vi "autofocus-view-calibration.vi"() -> ()   [LabVIEW 2014]
uses:
  autofocus-globals.vi
  TIRF/tirf-lock-globals.vi
panel:
  out "XY Graph":cluster{"Y":dbl[], "Y":dbl[]}[](graph)
  in  "Display":bool=TRUE
  out "Calibration curve":cluster{ext[], dbl[]}(graph)
  in  "?":bool
  in  "stop":bool
  out "Intensity 2":cluster{"X position":dbl, "Y position":dbl}(graph)
  out "Power Intensity":dbl(graph)
  # "Divide \nBy Sum"
  # "Raw"
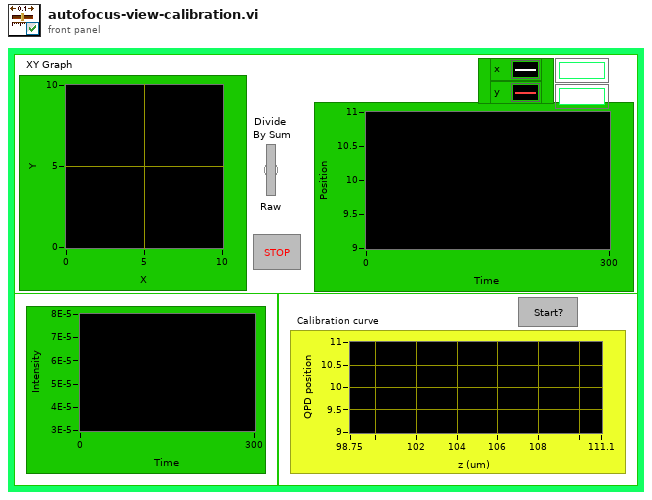
[diagram p1: front panel]
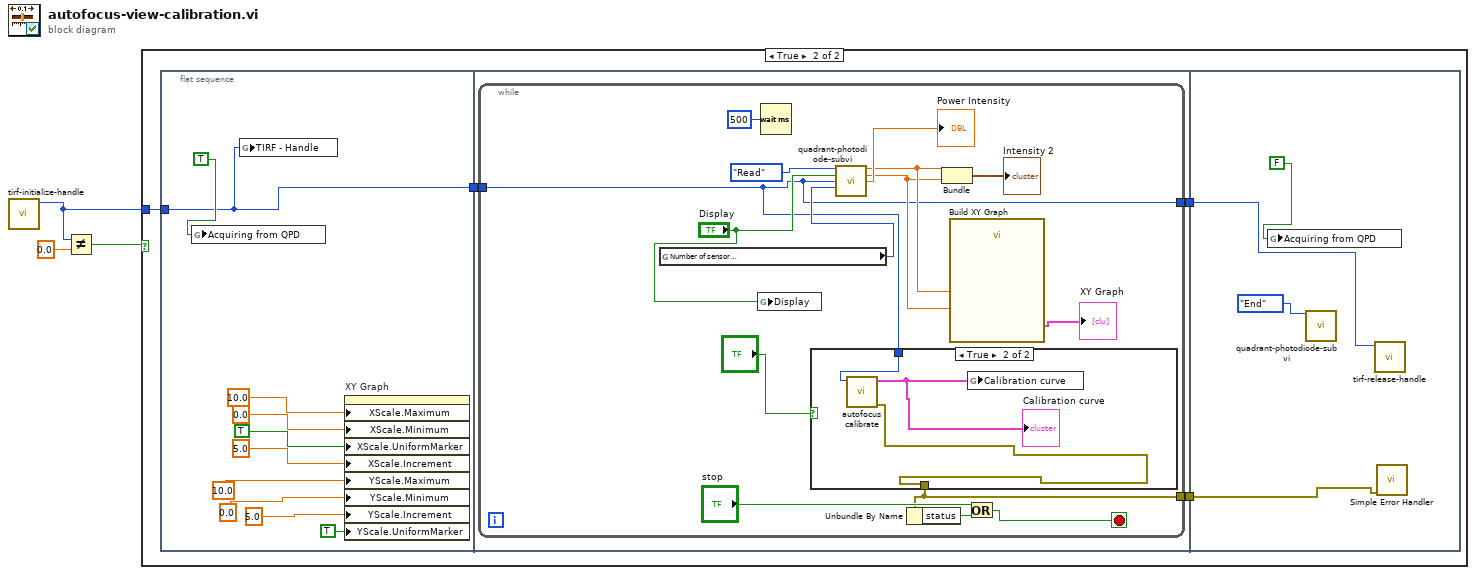
[diagram p0: block diagram]
diagram:
  n1 = call "tirf-initialize-handle.vi"() -> ("handle"=w1:i32)  [unwired: 11 in]
  n2 = Not Equal?(x=w1, y=0.0) -> (x != y?=w2:bool)
  n3 = case shown="True" w2 {
    tunnel: w1 -> [_ w5]
    frame False {
    }
    frame True {
      n4 = flat-sequence {
        tunnel: [w16] -> w6
        tunnel: w5 -> [w16]
        tunnel: [w20] -> w7
        tunnel: w6 -> [w19]
        tunnel: [w18] -> w4
        tunnel: w7 -> [w39]
        tunnel: w4 -> [w40]
        frame #0 {
          n5 = global write "autofocus-globals.vi" "Acquiring from QPD"(TRUE) -> ()
          n6 = global write "autofocus-globals.vi" "TIRF - Handle"(w16) -> ()
          n7 = property on="XY Graph" class="XYGraph (strict)"("XScale.Maximum"=10.0 ("X Scale.Range:Maximum"), "XScale.Minimum"=0.0 ("X Scale.Range:Minimum"), "XScale.UniformMarker"=TRUE ("X Scale.Uniform Marker Spacing?"), "XScale.Increment"=5.0 ("X Scale.Range:Increment"), "YScale.Maximum"=10.0 ("Y Scale.Range:Maximum"), "YScale.Minimum"=0.0 ("Y Scale.Range:Minimum"), "YScale.Increment"=5.0 ("Y Scale.Range:Increment"), "YScale.UniformMarker"=TRUE ("Y Scale.Uniform Marker Spacing?")) -> ()  [unwired: 2 in, 2 out]
        }
        frame #1 {
          n8 = while {
            tunnel: [w25] -> w20
            tunnel: w19 -> [w22]
            tunnel: [w22] -> w18
            stop <- w26 stop-if-true
            n9 = global read "autofocus-globals.vi" "Number of sensor\nreadings to average"() -> (w24:i32)
            n10 = global write "tirf-lock-globals.vi" "Display"("Display") -> ()
            n11 = Wait (ms)(milliseconds to wait=u32 500) -> ()  [unwired: 1 out]
            n12 = case shown="True" "?" {
              tunnel: [_ w37] -> w25
              tunnel: w22 -> [_ w38]
              frame False {
              }
              frame True {
                n13 = call "autofocus calibrate.vi"("Handle"=w38) -> ("Error Out"=w37:errorcluster, "Cal. curve"=w36:cluster{ext[], dbl[]})  [unwired: 7 in, 2 out]
                "Calibration curve" <- w36
                n14 = global write "autofocus-globals.vi" "Calibration curve"(w36) -> ()
              }
            }
            n15 = call "quadrant-photodiode-subvi.vi"("Mode"=enum16{"Start", "Read", "End"}."Read", "Display"="Display", "Handle"=w22, "Averages"=w24) -> ("coerced(x)"=w31:dbl, "coerced(y)"=w30:dbl, "Power (mw)"=→"Power Intensity":dbl)  [unwired: 9 in]
            n16 = Unbundle By Name(w25) -> ("status"=w27:bool)
            n17 = Bundle("coerced(x)"=w31, "coerced(y)"=w30) -> (→"Intensity 2":cluster{"coerced(x)":dbl, "coerced(y)":dbl})  [unwired: 1 in]
            n18 = call "Build XY Graph"("Y Input"=w30, "X Input"=w31) -> ("XY Graph"=→"XY Graph":cluster{"Y":dbl[], "Y":dbl[]}[])  [unwired: 3 in, 6 out]
            n19 = Or(x="stop", y=w27) -> (x .or. y?=w26:bool)
          }
        }
        frame #2 {
          n20 = global write "autofocus-globals.vi" "Acquiring from QPD"(FALSE) -> ()
          n21 = call "quadrant-photodiode-subvi.vi"("Mode"=enum16{"Start", "Read", "End"}."End") -> ()  [unwired: 12 in, 3 out]
          n22 = call "tirf-release-handle.vi"("handle"=w40) -> ()  [unwired: 11 in]
          n23 = call <vilib>:"Simple Error Handler.vi"("error in (no error)"=w39) -> ()  [unwired: 1 in, 8 out]
        }
      }
    }
  }
